vi "Test Mult.vi"(8 "error in (no error)":errorcluster, 11 "Test Case In":refnum<class "Rational Number Test.lvclass">) -> (0 "error out":errorcluster, 3 "Test Case Out":refnum<class "Rational Number Test.lvclass">)   [LabVIEW 2021, in "Rational Number Test.lvclass"]
uses:
  Rational Number Test.lvclass
  C:/Program Files (x86)/National Instruments/LabVIEW 2021/vi.lib/Astemes/LUnit/Test Case.lvclass
  <vilib>/Astemes/LUnit/Test Case.lvclass/Test Case.ctl
  4993e8ee-a06a-463a-9684-69129f64d5ce.vi
  <vilib>/Astemes/LUnit/Append Pass Result.vi
  <vilib>/Astemes/LUnit/Append Fail Result.vi
  <vilib>/Astemes/LUnit/Describe Comparison.vi
  <vilib>/Astemes/LUnit/Compare Variants.vi
  <vilib>/Astemes/LUnit/Variant to string.vi
  <vilib>/Utility/Data Type/Get Type Information.vi
  <vilib>/Utility/LVClass/Get LV Class Name.vi
  Rational Number Test.lvclass/Rational Number Test.ctl
  High Res Arithmetic/Rational Number.lvclass
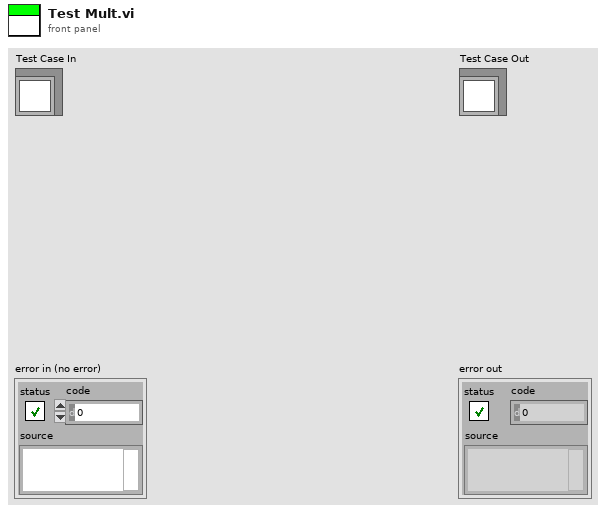
[diagram p1: front panel]
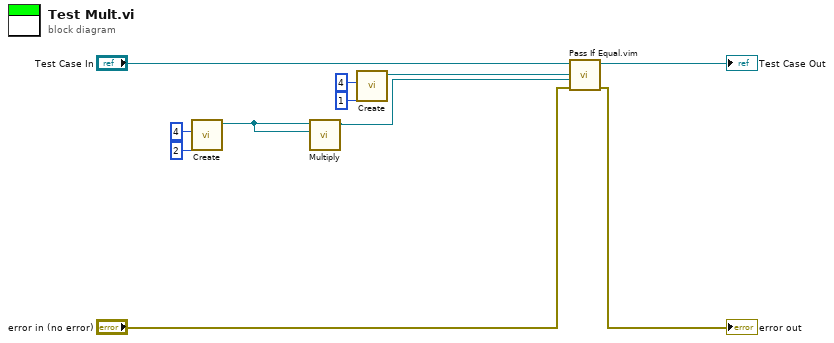
[diagram p0: block diagram]
diagram:
  n1 = call "Create.vi"("Denumerator"=i64 2, "Numerator"=i64 4 ("Integer Value")) -> ("Hi Res Arithm Test"=w1:refnum<class "Rational Number.lvclass">)  [unwired: 8 in, 1 out]
  n2 = call "Multiply.vi"("High Res Arithmetic 2"=w1, "High Res Arithmetic 1"=w1) -> ("High Res Arithmetic sum"=w4:refnum<class "Rational Number.lvclass">)  [unwired: 8 in, 1 out]
  n3 = call "Create.vi"("Denumerator"=i64 1, "Numerator"=i64 4 ("Integer Value")) -> ("Hi Res Arithm Test"=w5:refnum<class "Rational Number.lvclass">)  [unwired: 8 in, 1 out]
  n4 = call "Pass If Equal.vim"("error in (no error)"="error in (no error)", "Actual"=w4, "Expected"=w5, "LUnit Test Case In"="Test Case In") -> ("error out"=→"error out":errorcluster, "LUnit Test Case Out"=→"Test Case Out":refnum<class "Rational Number Test.lvclass">)  [unwired: 6 in]
